vi "Status.vi"(6 "Output Type":T1, 8 "error in (no error)":errorcluster, 11 "Git Implementation in":refnum<class "Git Implementation.lvclass">) -> (0 "error out":errorcluster, 2 "Status Message":string, 3 "Git Implementation out":refnum<class "Git Implementation.lvclass">)   [LabVIEW 2017, in "Git-LabVIEW.lvlib" / "Git Implementation.lvclass"]
doc: "Show the working tree status.\nFrom git-scm.com/docs/git-status:\nDisplays paths that have differences between the index file and the current HEAD commit, paths that have differences between the working tree and the index file, and paths in the working tree that are not tracked by Git (and are not ignored by gitignore).\nThe first are what you would commit by running git commit; the second and third are what you could commit by running git add before running git commit."
uses:
  Git Implementation.lvclass
  Output Type.ctl
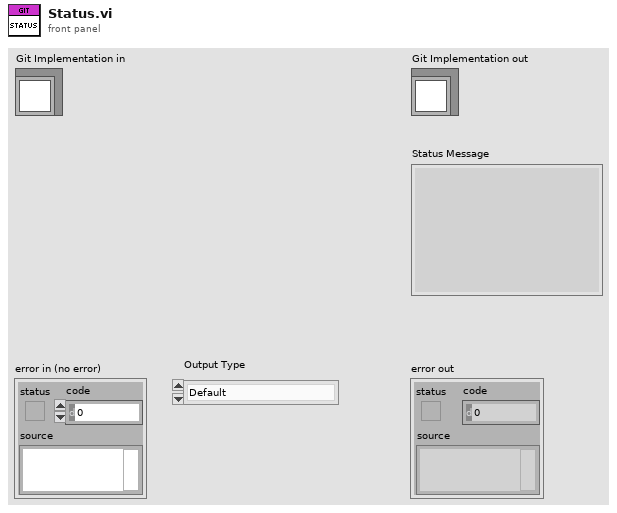
[diagram p1: front panel]
types:
  T1 = typedef "Git-LabVIEW.lvlib/Git Implementation.lvclass/Output Type.ctl" = enum16{"Default", "Porcelain-V1", "Porcelain-V2"}
  T2 = typedef "Git-LabVIEW.lvlib/Git Implementation.lvclass/CMD Return.ctl" = cluster{"StdOut":string, "StdErr":string, "Return Code":i32}
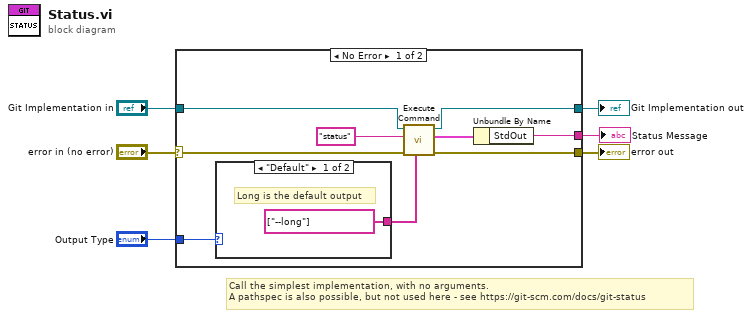
[diagram p0: block diagram]
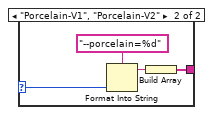
[diagram p2: hidden frame]
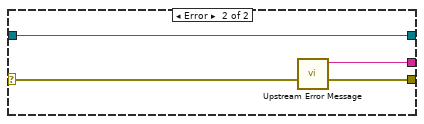
[diagram p3: hidden frame]
diagram:
  # "Call the simplest implementation, with no arguments.\nA pathspec is also possible, but not used here - see https://git-scm.com/docs/git-status"
  n1 = case shown="No Error" "error in (no error)" {
    selector: "error in (no error)" -> [w15 w23]
    tunnel: [w10 w23] -> w5
    tunnel: [w13 w22] -> w3
    tunnel: "Git Implementation in" -> [w14 w22]
    tunnel: [w9 w21] -> w2
    tunnel: "Output Type" -> [w8 _]
    frame No Error {
      n2 = case shown="\"Default\"" w8 {
        selector: w8 -> [_ w18]
        tunnel: [string[] ["--long"] w17] -> w7
        frame "Default" {
          # "Long is the default output"
        }
        frame "Porcelain-V1", "Porcelain-V2" {
          n3 = Format Into String(format string="--porcelain=%d", w18) -> (resulting string=w20:string)  [unwired: 2 in, 1 out]
          n4 = Build Array(w20) -> (w17:string[])
        }
      }
      n5 = call "Execute Command.vi"("Arguments"=w7, "error in (no error)"=w15, "Command"="status", "Git Implementation in"=w14) -> ("error out"=w10:errorcluster, "CMD Return"=w11:T2, "Git Implementation out"=w13:refnum<class "Git Implementation.lvclass">)  [unwired: 5 in]
      n6 = Unbundle By Name(w11) -> ("StdOut"=w9:string)
    }
    frame Error {
      n7 = call "Upstream Error Message.vi"() -> ("Upstream Error Message"=w21:string)  [unwired: 11 in]
    }
  }
  "error out" <- w5
  "Git Implementation out" <- w3
  "Status Message" <- w2
